vi "UDP Rx Process.vi"(10 "Parameters":variant, 11 "Process":refnum<class "Process.lvclass">) -> ()   [LabVIEW 2016, in "UDP-Custom-Device Engine.lvlib"]
uses:
  UDP-Custom-Device Engine.lvlib
  <vilib>/NI/NIVS Inline Async API/_VS Inline Async API/Process/Process.lvclass
  <vilib>/NI/NIVS Inline Async API/_VS Inline Async API/Process/Process.lvclass/Process.ctl
  <vilib>/NI/NIVS Inline Async API/_Data Access Engine/Access Type Classes/Write/Write.lvclass/Write.ctl
  <vilib>/NI/NIVS Inline Async API/_Data Access Engine/Data Access Engine/Methods/Write.Data.vi
  <vilib>/NI/NIVS Inline Async API/_VS Inline Async API/Process/Data Member Access/Read Data Access.vi
  <vilib>/NI/NIVS Inline Async API/_VS Inline Async API/Error Handling Process/SubVIs/Error.ConvertArray.vi
  <vilib>/NI/NIVS Inline Async API/_Data Access Engine/Access Type Classes/Write/Write.ProcessData.vi
  <vilib>/NI/NIVS Inline Async API/_Data Access Engine/Data Access Engine/Data Access Engine.lvclass
  <vilib>/NI Veristand/VeriStand Data/Library/VeriStand Data.lvlib
panel:
  out "Rx Packet":string
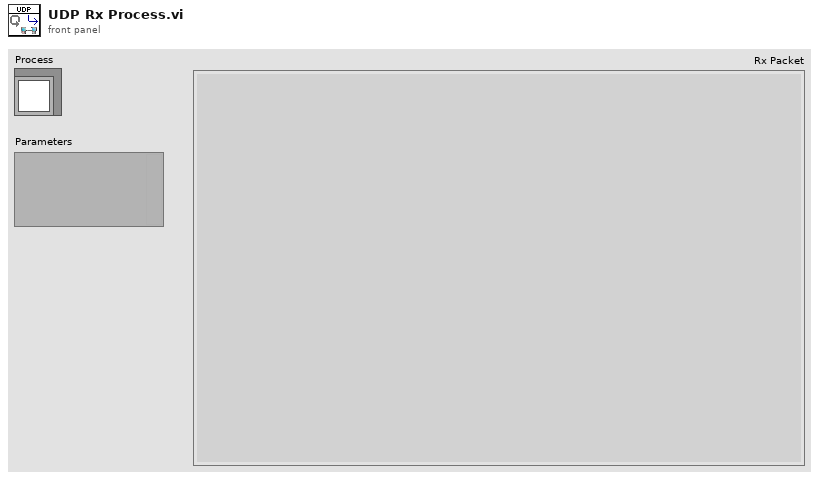
[diagram p1: front panel]
types:
  T1 = typedef "UDP-Custom-Device Engine.lvlib/Rx Loop Data.ctl" = cluster{"Packet Name":string, "Rx IP Address":string, "Packet ID":i32, "Timeout":i32, "Rx Port":i32, "Connection ID":refnum<k16>, "Rx FIFO Ref":T2, "Byte Order":enum16{"big-endian, network order", "native, host order", "little-endian"}, "Diagnostics En?":bool, "Header Info":bool[], "Channel Data Types":T3[], "Data Conversion":T4, "Header Details":T6}
  T2 = typedef "Data Access Engine.lvlib/Data Access Engine.lvclass/Write.DVR.ctl" = refnum<data-value>
  T3 = typedef "VeriStand Data.lvlib/Typedefs.Data Types.ctl" = enum16{"Boolean", "Single", "Double", "I8", "I16", "I32", "I64", "U8", "U16", "U32", "U64"}
  T4 = typedef "UDP-Custom-Device Engine.lvlib/Data Conversion Config.ctl" = cluster{"Byte Buffer":refnum<class "Byte Buffer.lvclass">, "Data Pointer":u64, "Channel Count":i32, "Mappings":T5[], "Static Header Payload":string, "Packet Count":dbl, "Packet Size":i32}
  T5 = typedef "VeriStand Data.lvlib/Byte Buffer.lvclass/Byte Buffer.Mapping.ctl" = cluster{"pointer":u64, "count":i32, "buffer offset":i32, "data type":T3}
  T6 = typedef "UDP-Custom-Device Shared.lvlib/Header Details.ctl" = cluster{"Packet Size":u16, "Protocol Revision":u8, "System Definition Version":u16, "Source Node Name":string, "Packet ID":u32, "Number of Channels":u32, "Static Header Size":u16, "Total Header Size":u16}
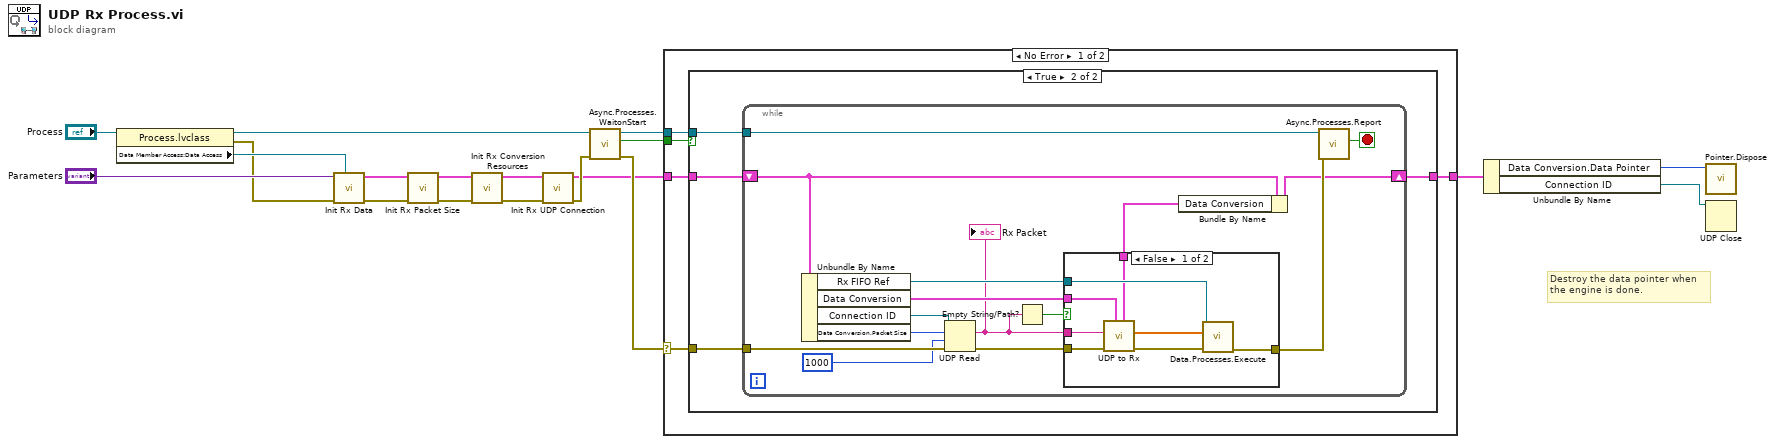
[diagram p0: block diagram]
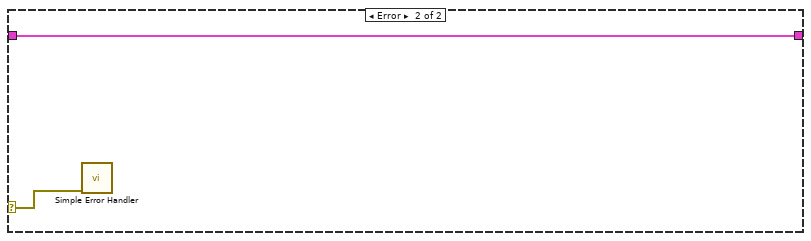
[diagram p4: hidden frame]
diagram:
  # "Destroy the data pointer when\nthe engine is done."
  n1 = property class="Process.lvclass"(reference="Process") -> (reference out=w19:refnum<class "Process.lvclass">, error out=w15:errorcluster, "Data Member Access:Data Access"=w16:refnum<class "Data Access Engine.lvclass">)  [unwired: 1 in]
  n2 = call "Init Rx Data.vi"("Data Access in"=w16, "error in (no error)"=w15, "Parameters"="Parameters") -> ("error out"=w4:errorcluster, "Rx Loop Data"=w6:T1)  [unwired: 6 in, 1 out]
  n3 = call "Init Rx Packet Size.vi"("error in (no error)"=w4, "Rx Loop Data"=w6) -> ("error out"=w3:errorcluster, "Rx Loop Data out"=w5:T1)  [unwired: 8 in]
  n4 = call "Init Rx Conversion Resources.vi"("error in (no error)"=w3, "Rx Loop Data"=w5) -> ("error out"=w7:errorcluster, "Rx Loop Data out"=w8:T1)  [unwired: 8 in]
  n5 = call "Init Rx UDP Connection.vi"("error in (no error)"=w7, "Rx Loop Data in"=w8) -> ("error out"=w11:errorcluster, "Rx Loop Data out"=w9:T1)  [unwired: 8 in]
  n6 = call <vilib>:"Async.Processes.WaitonStart.vi"("error in (no error)"=w11, "Process"=w19) -> ("error out"=w14:errorcluster, "Execute"=w12:bool, "Process out"=w13:refnum<class "Process.lvclass">)  [unwired: 7 in]
  n7 = case shown="No Error" w14 {
    selector: w14 -> [w22 w56]
    tunnel: w12 -> [w24 _]
    tunnel: w13 -> [w23 _]
    tunnel: w9 -> [w21 w55]
    tunnel: [w20 w55] -> w10
    frame No Error {
      n8 = case shown="True" w24 {
        tunnel: w22 -> [_ w28]
        tunnel: w23 -> [_ w29]
        tunnel: w21 -> [w25 w27]
        tunnel: [w25 w26] -> w20
        frame False {
        }
        frame True {
          n9 = while {
            tunnel: w28 -> [w41]
            tunnel: w29 -> [w44]
            shift-right: [w39] -> w26
            shift-left: w27 -> [w40]
            stop <- w43 stop-if-true
            n10 = Unbundle By Name(w40) -> ("Rx FIFO Ref"=w37:T2, "Data Conversion"=w36:T4, "Connection ID"=w38:refnum<k16>, "Data Conversion.Packet Size"=w34:i32)
            n11 = UDP Read(connection ID=w38, max size (548)=w34, timeout ms (25000)=1000, 8:w41) -> (data out=w31:string, error out=w33:errorcluster)  [unwired: 3 out]
            "Rx Packet" <- w31
            n12 = Empty String/Path?(string/path=w31) -> (empty?=w30:bool)
            n13 = case shown="False" w30 {
              tunnel: [w52 w54] -> w42
              tunnel: w37 -> [w51 _]
              tunnel: w31 -> [w50 _]
              tunnel: w36 -> [w49 w53]
              tunnel: [w48 w53] -> w35
              tunnel: w33 -> [w47 w54]
              frame False {
                n14 = call "UDP to Rx.vi"("Data Conversion"=w49, "error in (no error)"=w47, "Rx String"=w50) -> ("error out"=w46:errorcluster, "Rx Array"=w45:dbl[], "Data Conversion out"=w48:T4)  [unwired: 6 in]
                n15 = call-poly <vilib>:"Data.Processes.Execute.vi"("error in (no error)"=w46, "Values"=w45, "Ref"=w51) -> ("error out"=w52:errorcluster)  [unwired: 8 in]
              }
              frame True {
              }
            }
            n16 = Bundle By Name(cluster=w40, "Data Conversion"=w35) -> (w39:T1)
            n17 = call <vilib>:"Async.Processes.Report.vi"("Error"=w42, "Process in"=w44) -> ("Stop"=w43:bool)  [unwired: 8 in, 1 out]
          }
        }
      }
    }
    frame Error {
      n18 = call <vilib>:"Simple Error Handler.vi"("error in (no error)"=w56) -> ()  [unwired: 4 in, 5 out]
    }
  }
  n19 = Unbundle By Name(w10) -> ("Data Conversion.Data Pointer"=w2:u64, "Connection ID"=w1:refnum<k16>)
  n20 = call <vilib>:"Pointer.Dispose.vi"("pointer"=w2) -> ()  [unwired: 9 in, 2 out]
  n21 = UDP Close(connection ID=w1) -> ()  [unwired: 1 in, 2 out]
